vi "SignalFilterer.vi"(6 "Cutoff Frequency (Low End)":dbl min=0.0 max=22000.0 step=10.0, 7 "Cutoff Frequency (High End)":dbl, 9 "Sawtooth":dynamicdata(waveform), 10 "Filter Type":i32(knob) scale=0.0..2.0, 11 "Filter Toggle":bool) -> (2 "Filtered Signal":dynamicdata(waveform), 3 "Filter On":bool)   [LabVIEW 2022 SP3]
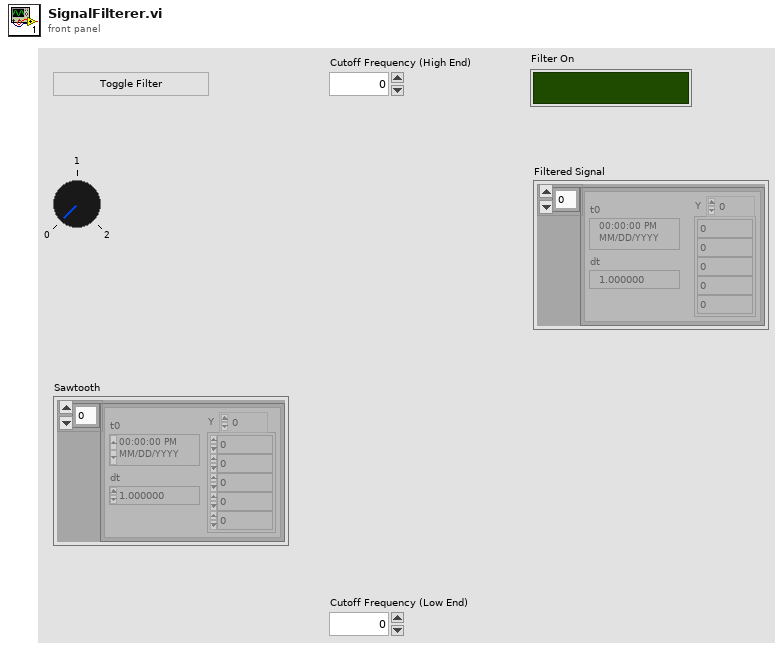
[diagram p1: front panel]
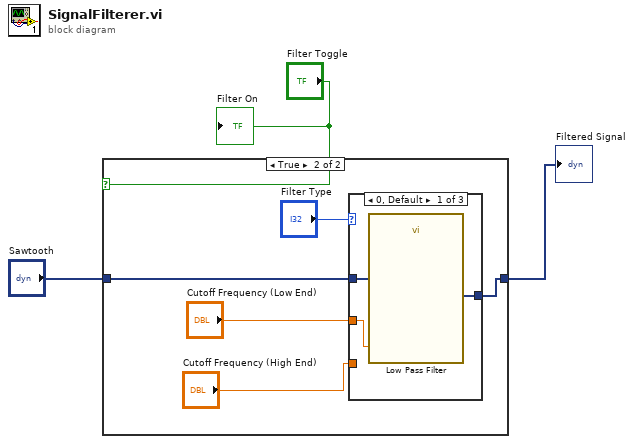
[diagram p0: block diagram]
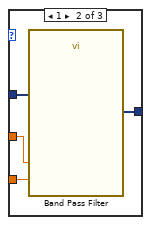
[diagram p3: hidden frame]
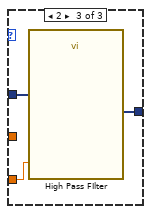
[diagram p4: hidden frame]
diagram:
  n1 = case shown="True" "Filter Toggle" {
    tunnel: "Sawtooth" -> [w4 w9]
    tunnel: [w4 w8] -> w3
    frame False {
    }
    frame True {
      n2 = case shown="0, Default" "Filter Type" {
        tunnel: "Cutoff Frequency (High End)" -> [_ w15 w19]
        tunnel: "Cutoff Frequency (Low End)" -> [w12 w16 _]
        tunnel: w9 -> [w11 w14 w18]
        tunnel: [w10 w13 w17] -> w8
        frame 0, Default {
          n3 = call "Low Pass Filter"("Lower Cut-Off"=w12, "Signal"=w11) -> ("Filtered Signal"=w10:dynamicdata)  [unwired: 8 in, 1 out]
        }
        frame 1 {
          n4 = call "Band Pass Filter"("Lower Cut-Off"=w16, "Upper Cut-Off"=w15, "Signal"=w14) -> ("Filtered Signal"=w13:dynamicdata)  [unwired: 7 in, 1 out]
        }
        frame 2 {
          n5 = call "High Pass FIlter"("Lower Cut-Off"=w19, "Signal"=w18) -> ("Filtered Signal"=w17:dynamicdata)  [unwired: 8 in, 1 out]
        }
      }
    }
  }
  "Filtered Signal" <- w3
  "Filter On" <- "Filter Toggle"
